vi "Sort Calibration.vi"(11 "Calibration (in)":dbl[][](array[numeric])) -> (0 "Abs Powers":dbl[](array[numeric]), 1 "Abs Energies":dbl[](array[numeric]), 3 "Calibration (out)":dbl[][](array[numeric]), 4 "Indexes":dbl[](array[numeric]))   [LabVIEW 2009]
uses:
  <vilib>/Analysis/NI_AALBase.lvlib
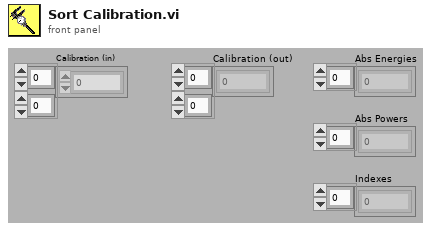
[diagram p1: front panel]
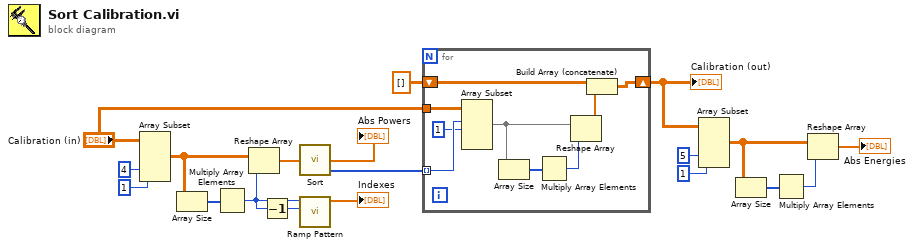
[diagram p0: block diagram]
diagram:
  n1 = Array Subset(array="Calibration (in)", index (col)=4 ("index"), length (col)=1 ("length")) -> (w3:dbl[][])  [unwired: 2 in]
  n2 = Array Size(array=w3) -> (size(s)=w4:i32[])
  n3 = Multiply Array Elements(1:w4) -> (0:w6:i32)
  n4 = Reshape Array(w3, w6) -> (w8:dbl[])
  n5 = Decrement(x=w6) -> (x-1=w5:i32)
  n6 = call "Sort.vi"("Array"=w8) -> ("Indices"=w10:i32[], "Sorted array"=→"Abs Powers":dbl[])  [unwired: 3 in]
  n7 = call <vilib>:"Ramp Pattern.vi"("end"=w5, "samples"=w6) -> ("Ramp Pattern"=→"Indexes":dbl[])  [unwired: 8 in, 1 out]
  n8 = for {
    tunnel: "Calibration (in)" -> [w25]
    tunnel: w10 -> [w24] mode=indexing
    shift-right: [w20] -> w18
    shift-left: dbl[][] [] -> [w21]
    n9 = Array Subset(array=w25, index (row)=w24, length (row)=1 ("length")) -> (w26:dbl[][])  [unwired: 2 in]
    n10 = Array Size(array=w26) -> (size(s)=w27:i32[])
    n11 = Multiply Array Elements(1:w27) -> (0:w28:i32)
    n12 = Reshape Array(w26, w28) -> (w22:dbl[])
    n13 = Build Array (concatenate)(w21, w22) -> (w20:dbl[][])
  }
  "Calibration (out)" <- w18
  n14 = Array Subset(array=w18, index (col)=5 ("index"), length (col)=1 ("length")) -> (w16:dbl[][])  [unwired: 2 in]
  n15 = Array Size(array=w16) -> (size(s)=w15:i32[])
  n16 = Multiply Array Elements(1:w15) -> (0:w14:i32)
  n17 = Reshape Array(w16, w14) -> (→"Abs Energies":dbl[])
